vi "Offset.vi"(7 "Raw Data Waveform":T1, 10 "Offset":i32, 11 "((Pointer))":refnum<class "((Pointer)).lvclass">) -> (3 "((Pointer)) Out":refnum<class "((Pointer)).lvclass">)   [LabVIEW 2016, in "((Pointer)).lvclass"]
uses:
  ((Pointer)).lvclass
  Universal Controls/Waveform_Data.ctl
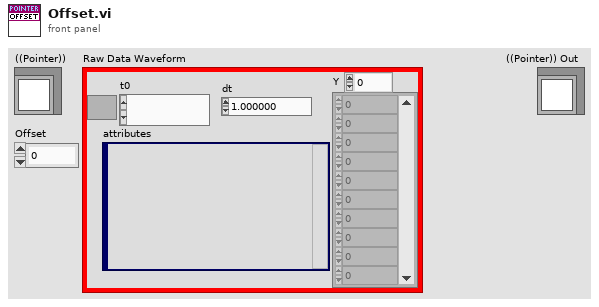
[diagram p1: front panel]
types:
  T1 = typedef "Waveform_Data.ctl" = waveform(dbl)
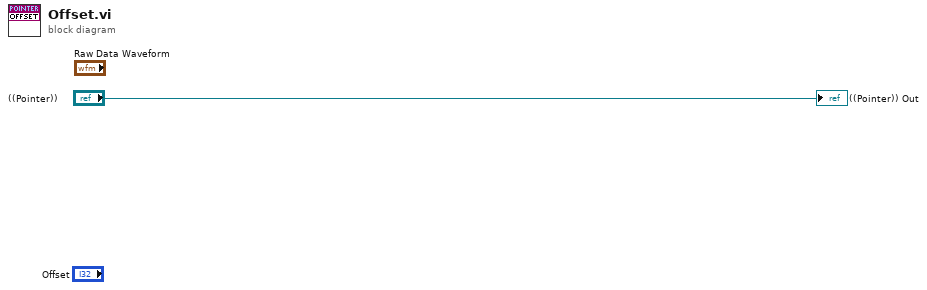
[diagram p0: block diagram]
diagram:
  "((Pointer)) Out" <- "((Pointer))"
